vi "manualGainDivisor.vi"(10 "Use DDS display equivalent?":bool, 11 "Gain Divisor (number of bits to shift)":u8) -> (2 "Gain Denominator":u8, 3 "Gain divisor string out":string)   [LabVIEW 2012, in "DDS9954_v2013.lvlib"]
uses:
  DDS9954_v2013.lvlib
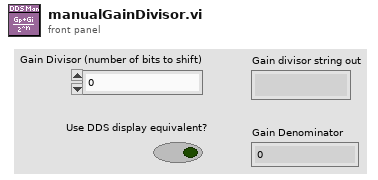
[diagram p1: front panel]
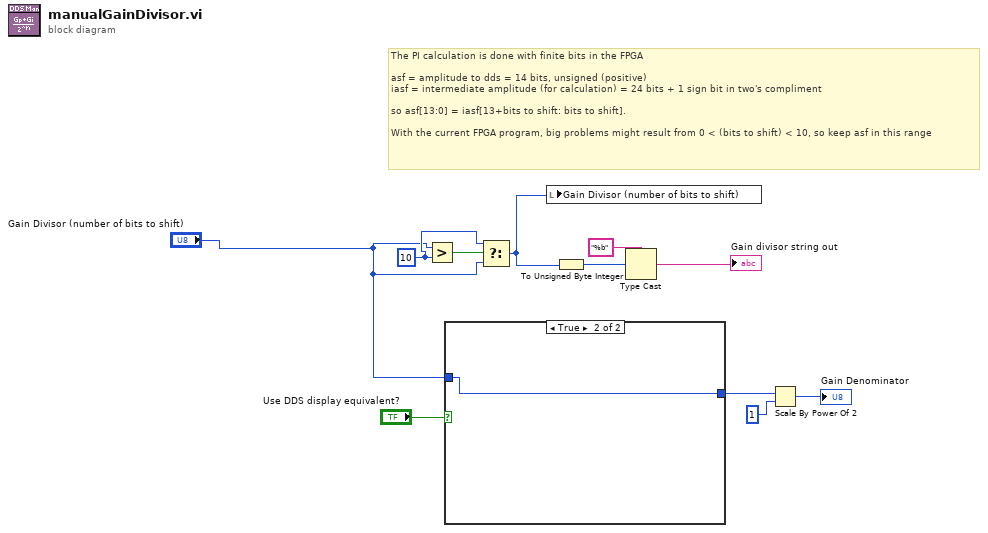
[diagram p0: block diagram]
diagram:
  w3 = u8 10 ("y")
  # "The PI calculation is done with finite bits in the FPGA\n\nasf = amplitude to dds = 14 bits, unsigned (positive)\niasf = intermediate amplitude (for calculation) = 24 bits + 1 sign bit in two's compliment\n\nso asf[13:0] = iasf[13+bits to shift: bits to shift].\n\nWith the current FPGA program, big problems might result from 0 < (bits to shift) < 10, so keep asf in this range"
  n1 = Greater?(x="Gain Divisor (number of bits to shift)", y=w3) -> (0:w4:bool)
  n2 = case shown="True" "Use DDS display equivalent?" {
    tunnel: "Gain Divisor (number of bits to shift)" -> [w12 w13]
    tunnel: [w12 w13] -> w7
    frame False {
    }
    frame True {
    }
  }
  n3 = Select(t=w3, s=w4, f="Gain Divisor (number of bits to shift)") -> (s? t:f=w1:u8)
  n4 = local write "Gain Divisor (number of bits to shift)"(w1) -> ()
  n5 = To Unsigned Byte Integer(number=w1) -> (unsigned 8bit integer=w11:u8)
  n6 = Type Cast(type="%b", x=w11) -> (*(type *) &x=→"Gain divisor string out":string)
  n7 = Scale By Power Of 2(n=w7, x=u8 1) -> (x*2^n=→"Gain Denominator":u8)
